vi "barrierOrManMark.vi"(8 "error in (no error)":errorcluster, 9 "Number of Defenders\nWithout Duelist":i32, 10 "Game":refnum<class "Game.lvclass">, 11 "DefendAreaSkill in":refnum<class "DefendAreaSkill.lvclass">) -> (0 "error out":errorcluster, 1 "Enemy position\nto mark":dbl[](array[numeric]), 2 "Type of Defense Barrier":enum16{"Barreira", "Manmark"}(ring), 3 "DefendAreaSkill out":refnum<class "DefendAreaSkill.lvclass">)   [LabVIEW 2023, in "DefendAreaSkill.lvclass"]
uses:
  DefendAreaSkill.lvclass
  Game_class/Game.lvclass
  Game_class/Game.lvclass/Game.ctl
  Team_class/Team.lvclass/Team.ctl
  Parameters_class/Parameters.lvclass/Parameters.ctl
  Object_class/Object.lvclass/Object.ctl
  Object_class/Read x.vi
  Object_class/Read y.vi
  Team_class/Read RobotRef.vi
  Game_class/Read Utilities.lvclass.vi
  Game_class/Read EnemyRef.vi
  Game_class/Read Parameters.lvclass.vi
  Game_class/Read OffensiveTeam.vi
  Game_class/Read BallRef.vi
  Parameters_class/Read AttakingOurselves.vi
  Enemy_class/Enemy.lvclass
  Ally_class/Ally.lvclass
  Robot_class/Robot.lvclass
  Utilities_class/Utilities.lvclass
  Parameters_class/Parameters.lvclass
  Ball_class/Ball.lvclass
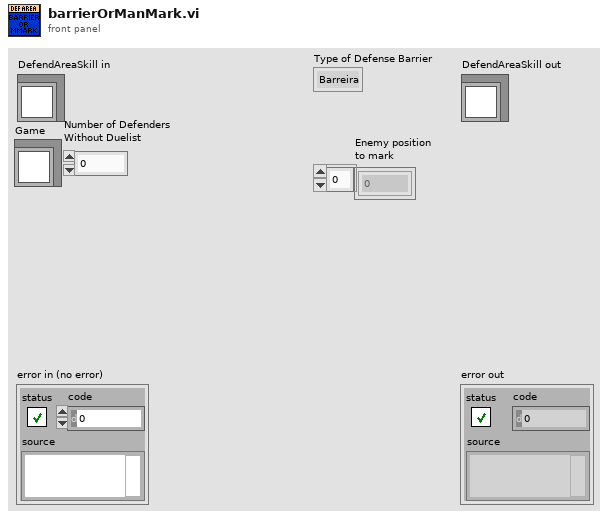
[diagram p1: front panel]
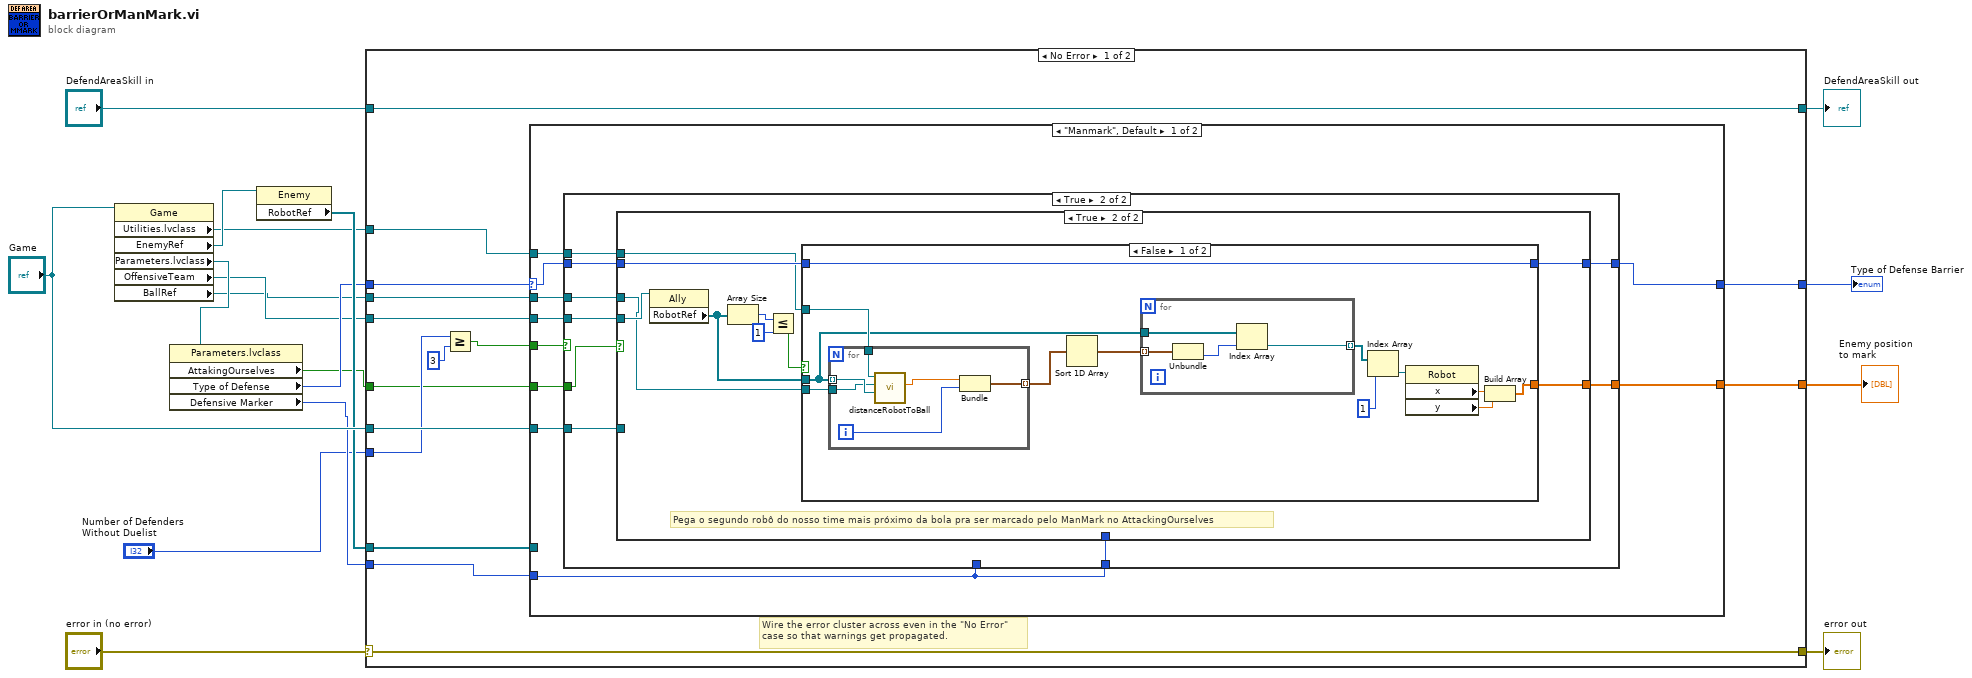
[diagram p0: block diagram]
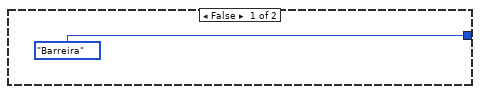
[diagram p2: hidden frame]
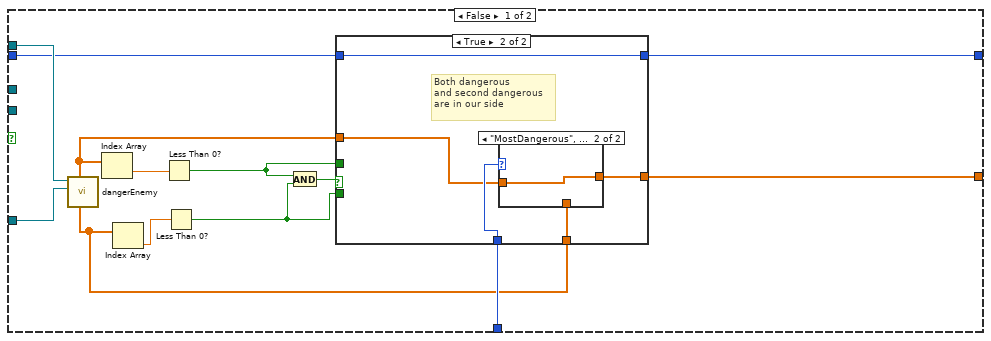
[diagram p3: hidden frame]
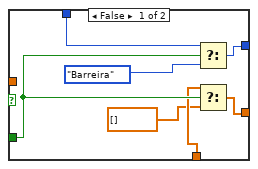
[diagram p5: hidden frame]
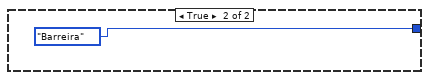
[diagram p7: hidden frame]
diagram:
  n1 = property class="Game"(reference="Game") -> ("Utilities.lvclass"=w2:refnum<class "Utilities.lvclass">, "EnemyRef"=w12:refnum<class "Enemy.lvclass">, "Parameters.lvclass"=w6:refnum<class "Parameters.lvclass">, "OffensiveTeam"=w3:refnum<class "Ally.lvclass">, "BallRef"=w1:refnum<class "Ball.lvclass">)  [unwired: 1 in, 2 out]
  n2 = property class="Parameters.lvclass"(reference=w6) -> ("AttakingOurselves"=w4:bool, "Type of Defense"=w8:enum16{"Barreira", "Manmark"}, "Defensive Marker"=w9:enum16{"SecondMostDangerous", "MostDangerous"})  [unwired: 1 in, 2 out]
  n3 = property class="Enemy"(reference=w12) -> ("RobotRef"=w11:refnum<class "Robot.lvclass">[])  [unwired: 1 in, 2 out]
  n4 = case shown="No Error" "error in (no error)" {
    selector: "error in (no error)" -> [w31 w125]
    tunnel: [w31 w125] -> w16
    tunnel: [w32 w124] -> w14
    tunnel: "DefendAreaSkill in" -> [w32 w124]
    tunnel: w8 -> [w30 w123]
    tunnel: [w29 w123] -> w7
    tunnel: "Game" -> [w28 _]
    tunnel: w11 -> [w27 _]
    tunnel: w9 -> [w26 _]
    tunnel: [w25 _] -> w10
    tunnel: "Number of Defenders\nWithout Duelist" -> [w24 _]
    tunnel: w4 -> [w21 _]
    tunnel: w3 -> [w20 _]
    tunnel: w2 -> [w19 _]
    tunnel: w1 -> [w18 _]
    frame No Error {
      # "Wire the error cluster across even in the \"No Error\"\ncase so that warnings get propagated."
      n5 = Greater Or Equal?(x=w24, y=3) -> (x >= y?=w22:bool)
      n6 = case shown="\"Manmark\", Default" w30 {
        selector: w30 -> [w38 w122]
        tunnel: [w41 w122] -> w29
        tunnel: w19 -> [w40 _]
        tunnel: w28 -> [w42 _]
        tunnel: w27 -> [_ _]
        tunnel: w26 -> [w37 _]
        tunnel: [w39 _] -> w25
        tunnel: w22 -> [w36 _]
        tunnel: w21 -> [w35 _]
        tunnel: w20 -> [w34 _]
        tunnel: w18 -> [w33 _]
        frame "Manmark", Default {
          n7 = case shown="True" w36 {
            tunnel: w42 -> [_ w52]
            tunnel: [enum16{"Barreira", "Manmark"}."Barreira" ("Type of Defense Barrier") w51] -> w41
            tunnel: w37 -> [_ w50]
            tunnel: w40 -> [_ w49]
            tunnel: [_ w48] -> w39
            tunnel: w38 -> [_ w47]
            tunnel: w37 -> [_ _]
            tunnel: w35 -> [_ w46]
            tunnel: w34 -> [_ w45]
            tunnel: w33 -> [_ w44]
            frame False {
            }
            frame True {
              n8 = case shown="True" w46 {
                tunnel: w52 -> [w65 _]
                tunnel: [w61 w94] -> w51
                tunnel: w50 -> [w60 _]
                tunnel: w49 -> [w57 w91]
                tunnel: [w56 w90] -> w48
                tunnel: w47 -> [w53 w93]
                tunnel: w45 -> [_ w98]
                tunnel: w44 -> [_ w89]
                frame False {
                  n9 = call "dangerEnemy.vi"("Game"=w65, "Utilities in"=w57) -> ("Pos do segundo inimigo\nperigoso"=w54:dbl[], "Pos do inimigo\nmais perigoso"=w55:dbl[])  [unwired: 3 in, 5 out]
                  n10 = Index Array(array=w55) -> (element=w64:dbl)  [unwired: 1 in]
                  n11 = Index Array(array=w54) -> (element=w63:dbl)  [unwired: 1 in]
                  n12 = Less Than 0?(x=w64) -> (x < 0?=w59:bool)
                  n13 = Less Than 0?(x=w63) -> (x < 0?=w58:bool)
                  n14 = And(x=w59, y=w58) -> (x .and. y?=w62:bool)
                  n15 = case shown="True" w62 {
                    tunnel: [w71 w82] -> w61
                    tunnel: w60 -> [_ w86]
                    tunnel: w59 -> [w72 _]
                    tunnel: w58 -> [w70 _]
                    tunnel: [w69 w85] -> w56
                    tunnel: w55 -> [w68 w84]
                    tunnel: w54 -> [w67 w83]
                    tunnel: w53 -> [w66 w82]
                    frame False {
                      n16 = case shown="True" w72 {
                        tunnel: [w77 w80] -> w71
                        tunnel: w70 -> [w79 _]
                        tunnel: [w75 w81] -> w69
                        tunnel: w68 -> [_ w81]
                        tunnel: w67 -> [w76 _]
                        tunnel: w66 -> [w78 w80]
                        frame False {
                          n17 = Select(t=w78, s=w79, f=enum16{"Barreira", "Manmark"}."Barreira" ("Type of Defense Barrier")) -> (s? t:f=w77:enum16{"Barreira", "Manmark"})
                          n18 = Select(t=w76, s=w79, f=dbl[] []) -> (s? t:f=w75:dbl[])
                        }
                        frame True {
                          # "Just dangerous is in our side"
                        }
                      }
                    }
                    frame True {
                      # "Both dangerous\nand second dangerous\nare in our side"
                      n19 = case shown="\"MostDangerous\", Default" w86 {
                        tunnel: [w87 w88] -> w85
                        tunnel: w84 -> [_ w88]
                        tunnel: w83 -> [w87 _]
                        frame "SecondMostDangerous" {
                        }
                        frame "MostDangerous", Default {
                        }
                      }
                    }
                  }
                }
                frame True {
                  # "Pega o segundo robô do nosso time mais próximo da bola pra ser marcado pelo ManMark no AttackingOurselves"
                  n20 = property class="Ally"(reference=w98) -> ("RobotRef"=w92:refnum<class "Robot.lvclass">[])  [unwired: 1 in, 2 out]
                  n21 = Array Size(array=w92) -> (size(s)=w97:i32)
                  n22 = Less Or Equal?(x=w97, y=1) -> (x <= y?=w95:bool)
                  n23 = case shown="False" w95 {
                    tunnel: [w110 enum16{"Barreira", "Manmark"}."Barreira" ("Type of Defense Barrier")] -> w94
                    tunnel: w93 -> [w110 _]
                    tunnel: w92 -> [w106 _]
                    tunnel: w91 -> [w107 _]
                    tunnel: [w100 _] -> w90
                    tunnel: w89 -> [w99 _]
                    frame False {
                      n24 = for {
                        tunnel: w106 -> [w117] mode=indexing
                        tunnel: [w119] -> w108 mode=indexing
                        tunnel: w107 -> [w118]
                        tunnel: w99 -> [w115]
                        i -> [w120]
                        n25 = call "distanceRobotToBall.vi"("Robot"=w117, "Ball"=w115, "Utilities in"=w118) -> ("Distance Robot To Ball"=w116:dbl)  [unwired: 6 in, 2 out]
                        n26 = Bundle("Distance Robot To Ball"=w116, w120) -> (w119:cluster{"Distance Robot To Ball":dbl, i32})  [unwired: 1 in]
                      }
                      n27 = Sort 1D Array(array=w108) -> (sorted array=w109:cluster{"Distance Robot To Ball":dbl, i32}[])
                      n28 = for {
                        tunnel: w109 -> [w113] mode=indexing
                        tunnel: w106 -> [w114]
                        tunnel: [w111] -> w105 mode=indexing
                        n29 = Unbundle(w113) -> (w112:i32)  [unwired: 1 out]
                        n30 = Index Array(array=w114, index=w112) -> (element=w111:refnum<class "Robot.lvclass">)
                      }
                      n31 = Index Array(array=w105, index=1) -> (element=w103:refnum<class "Robot.lvclass">)
                      n32 = property class="Robot"(reference=w103) -> ("x"=w102:dbl, "y"=w101:dbl)  [unwired: 1 in, 2 out]
                      n33 = Build Array(w102, w101) -> (w100:dbl[])
                    }
                    frame True {
                    }
                  }
                }
              }
            }
          }
        }
        frame "Barreira" {
        }
      }
    }
    frame Error {
    }
  }
  "error out" <- w16
  "DefendAreaSkill out" <- w14
  "Enemy position\nto mark" <- w10
  "Type of Defense Barrier" <- w7
